vi "get_unpack_len.vi"(3 "error in":errorcluster, 5 "u":u64) -> (0 "error out":errorcluster, 1 "len":u32, 2 "u out":u64)   [LabVIEW 2019, in "msgunpack.lvlib"]
doc: "Returns the number of bytes in the internal buffer remaining to be unpacked."
uses:
  msgunpack.lvlib
  msgpackalt.dll
panel:
  # "msgpack"
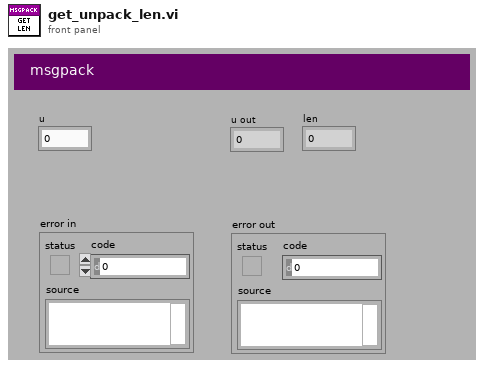
[diagram p1: front panel]
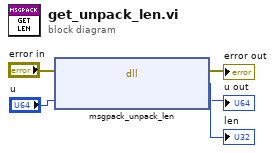
[diagram p0: block diagram]
diagram:
  n1 = dll-call lib="C:/Users/Patrick/Documents/GitHub/Instrument-Framework/lvsrc/SMOs/JSON-RPC-2019/lv-venv/lv.lib/vi.lib/addons/msgpack/msgpackalt.dll" fn="msgpack_unpack_len"(error in="error in", "p"="u") -> (error out=→"error out":errorcluster, "return type"=→"len":u32, "p"=→"u out":u64)  [unwired: 2 in, 1 out]
